vi "_TCP Msg Write_tester.vi"(7 "RT":bool, 8 "error in":errorcluster, 9 "timeout ms (10000)":i32=10000, 10 "Packet Info In":T1={"Packet Signature"="", "Sequence Number"=0, "Command"=enum."xml Set LC Input Logic", "Data Message Size"=0, "Data Message Size"="", "Data Message"="", "Error Message Size"=0, "Error Message Size"="", "Error Message"="", "Checksum"=0, "Error Message"={"status"=FALSE, "code"=0, "source"=""}, "Command ID"=""}, 11 "connection ID In":refnum<k5>) -> (0 "error out":errorcluster, 2 "Packet Info In Out":T1={"Packet Signature"="", "Sequence Number"=0, "Command"=enum."Get Info", "Data Message Size"=0, "Data Message Size"="", "Data Message"="", "Error Message Size"=0, "Error Message Size"="", "Error Message"="", "Checksum"=0, "Error Message"={"status"=FALSE, "code"=0, "source"=""}, "Command ID"=""}, 3 "connection ID out":refnum<k5>)   [LabVIEW 2015]
doc: "Writes a package of data to a remote computer via TCP/IP. The VI appends an ID number to each packet. This ID number is used by the Comm TCP Read VI to parse the packet using the meta data. This technique allows appending variable name and type to each packet for ease of use while minimizing the transmission overhead.\n\nThe data must be passed in as a String. The user is responsible for casting or flattening the desired data into a String before passing it to this VI. \n\n* Use the same method for converting to/from String on both the Read and Write functions. For example, if you use the 'Cast' primitive to convert the data into a String, make sure that the 'Cast' primitive is used on the receiving side to convert the data from String to its original form."
uses:
  Type/TCP Packet Info.ctl
  Type/_RT Command.ctl
  Type/TCP Packet Parsing State Machine.ctl
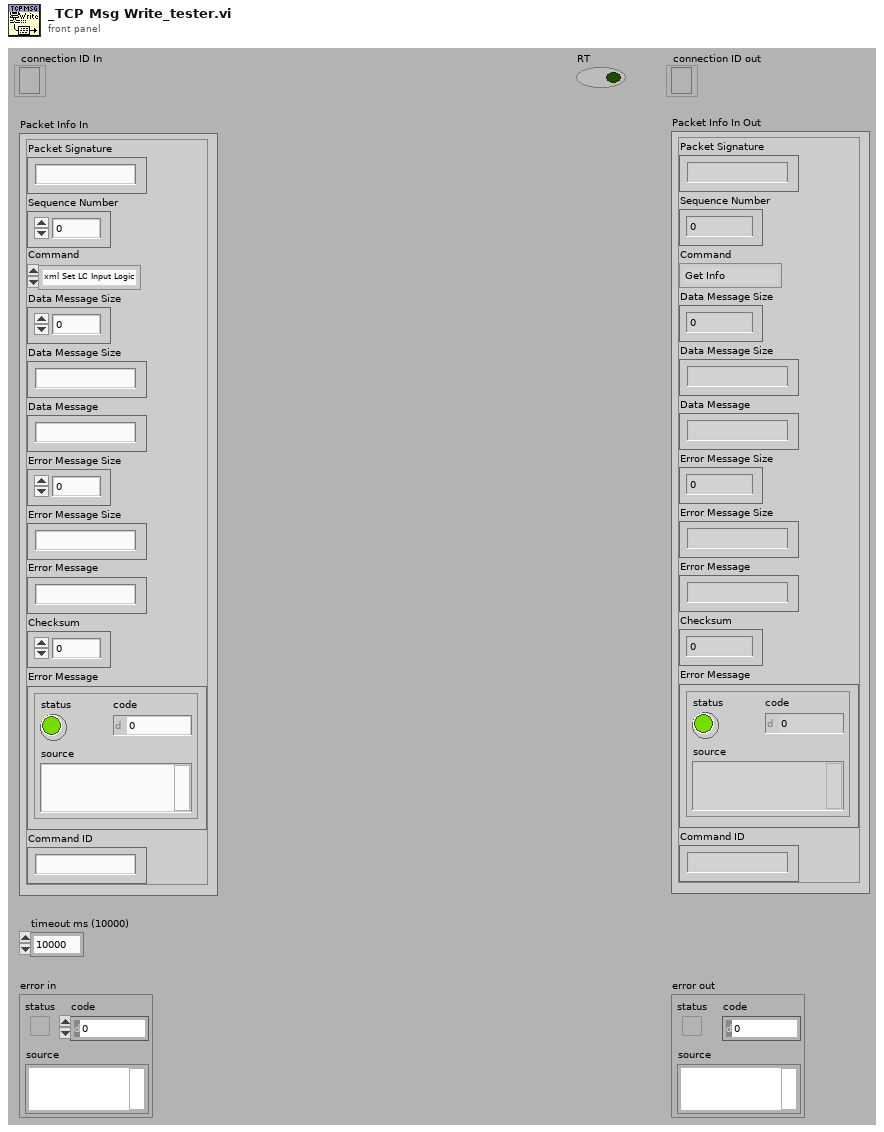
[diagram p1: front panel]
types:
  T1 = typedef "TCP Packet Info.ctl" = cluster{"Packet Signature":string, "Sequence Number":i32, "Command":T2, "Data Message Size":u32, "Data Message Size":string, "Data Message":string, "Error Message Size":u32, "Error Message Size":string, "Error Message":string, "Checksum":u32, "Error Message":errorcluster, "Command ID":string}
  T2 = typedef "_RT Command.ctl" = enum16{"xml Start Run", "xml Start Actual Run", "xml Stop Run", "xml Runtime Update", "xml Get Status", "xml Get Table", "xml Set Table", "xml Get Configuration", "xml System Status", "xml Set LC Input Logic", "xml Get Data", "xml Get Info", "Start", "StartActualRun", "Stop", "Runtime Update", "Get Data", "Get Info", "Get Status", "Get Param", "Get Config", "Get Table", "Read ADC", "Set Oscillator", "Update Config", "Update Table", "Set All Pol", "Set Pol and DC", "Set Max Mass", "Toggle RP", "Toggle EL", "Set PIC", "Initialize Turbo", "Send Turbo Comm", "Close Turbo", "P1", "P2", "P3", "Send Serial", "Set LC Out", "Get LC In", "Read VAC", "Test Table", "Toggle Power", "Get Startup", "Set Startup", "Get ADC Table", "Set ADC Table", "Get Brief Status", "Get Detail Status", "Auxiliary Update", "Set CC Logics", "Set CC Input Logics", "Ignore Error", "invalid"}
  T3 = typedef "TCP Packet Parsing State Machine.ctl" = enum16{"Packet Signature", "Sequence Number", "Command ID", "Data Message Size", "Data Message", "Error Message Size", "Error Message", "Checksum", "Invalid Packet Structure"}
  T4 = enum16{"big-endian, network order", "native, host order", "little-endian"}
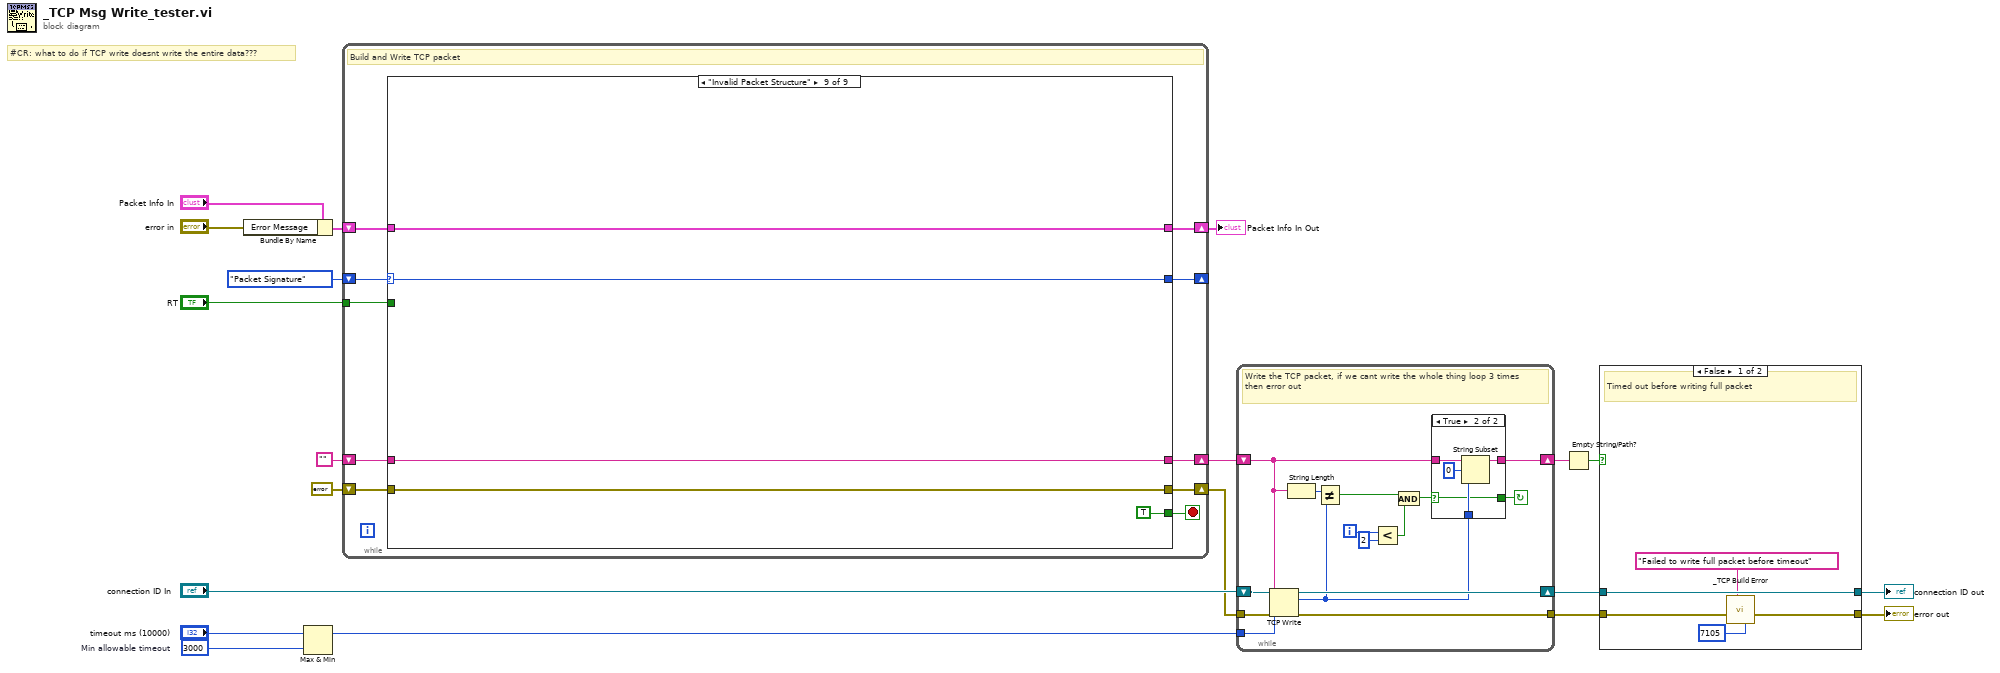
[diagram p0: block diagram]
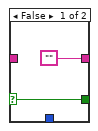
[diagram p3: hidden frame]
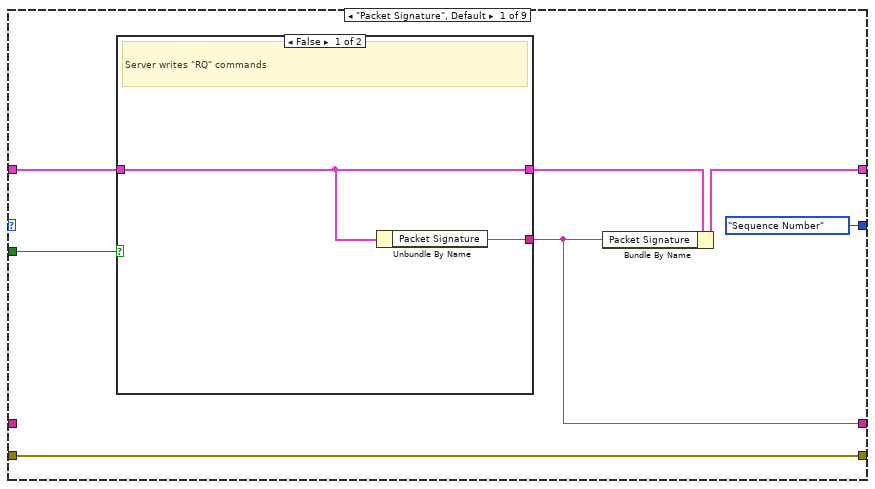
[diagram p4: hidden frame]
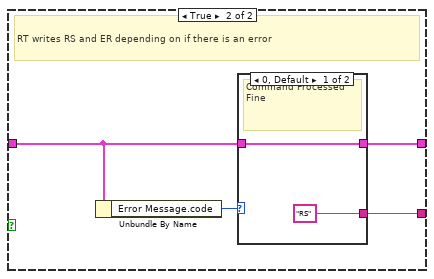
[diagram p5: hidden frame]
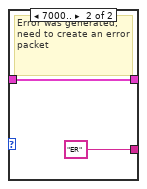
[diagram p6: hidden frame]
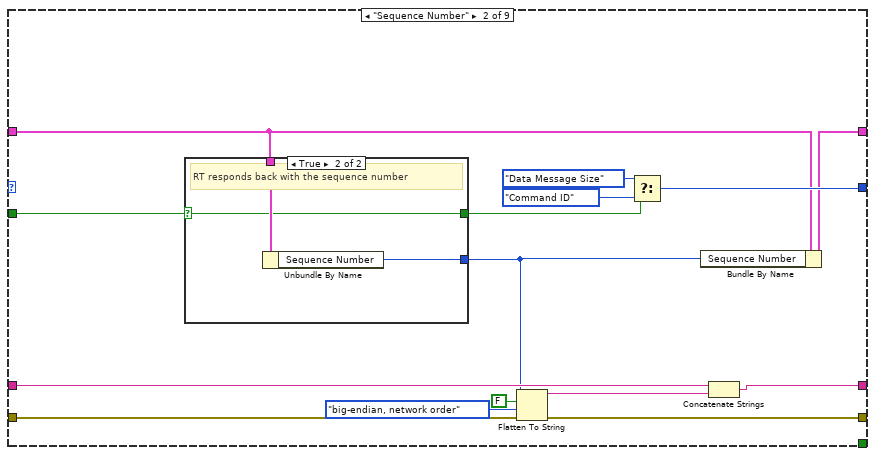
[diagram p7: hidden frame]
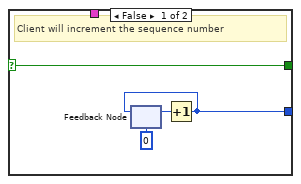
[diagram p8: hidden frame]
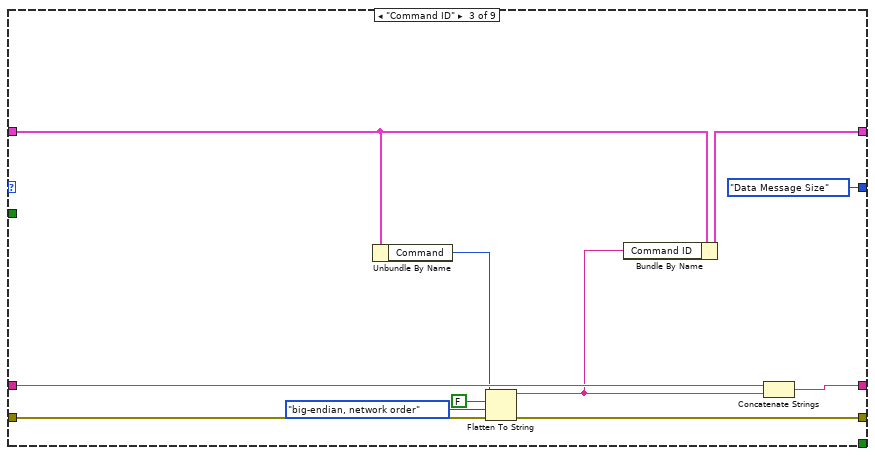
[diagram p9: hidden frame]
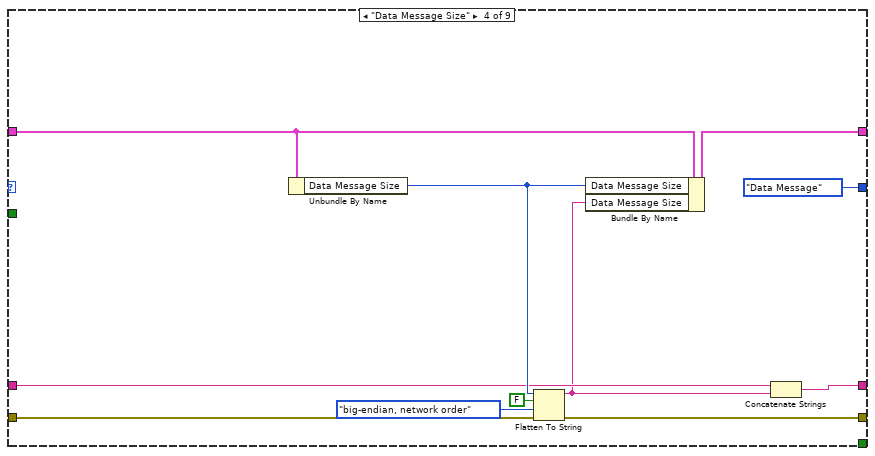
[diagram p10: hidden frame]
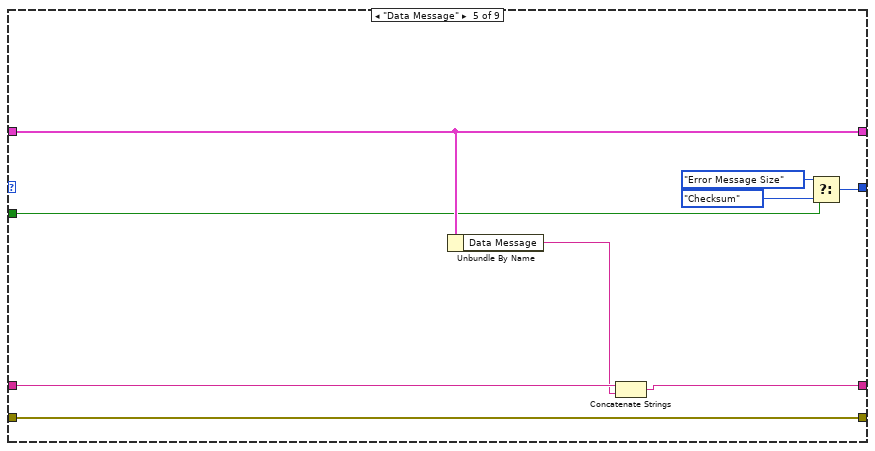
[diagram p11: hidden frame]
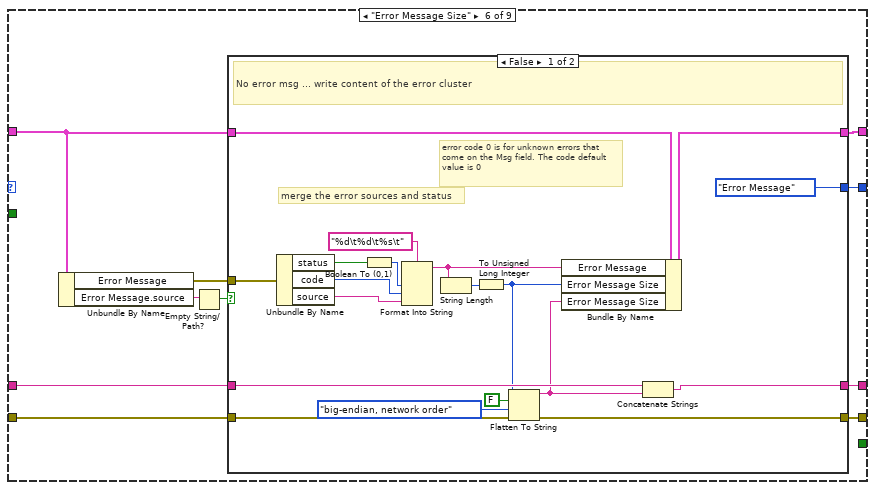
[diagram p12: hidden frame]
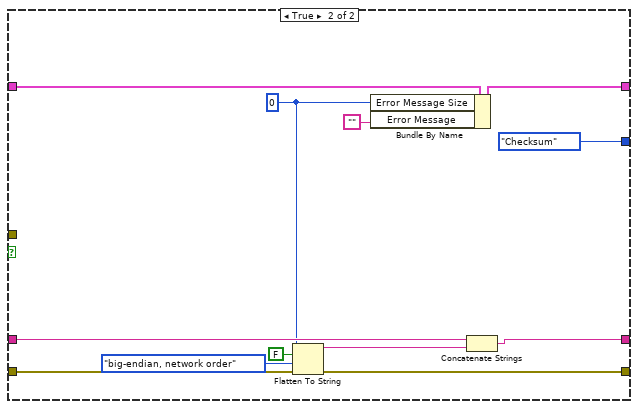
[diagram p13: hidden frame]
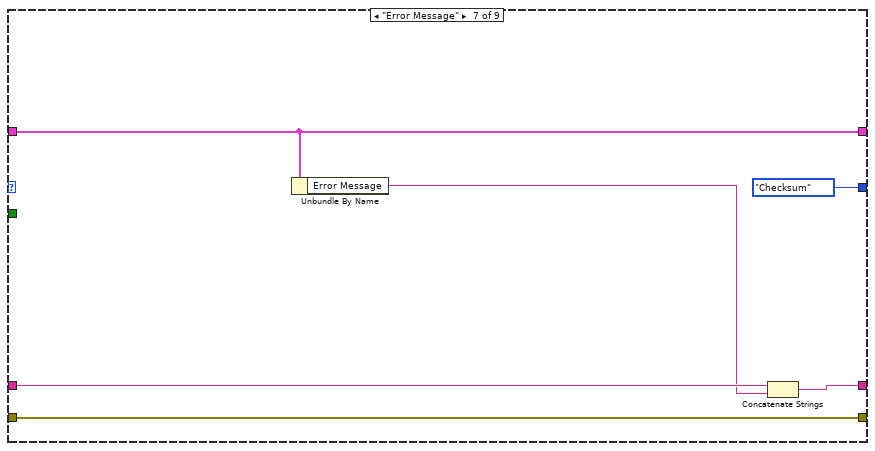
[diagram p14: hidden frame]
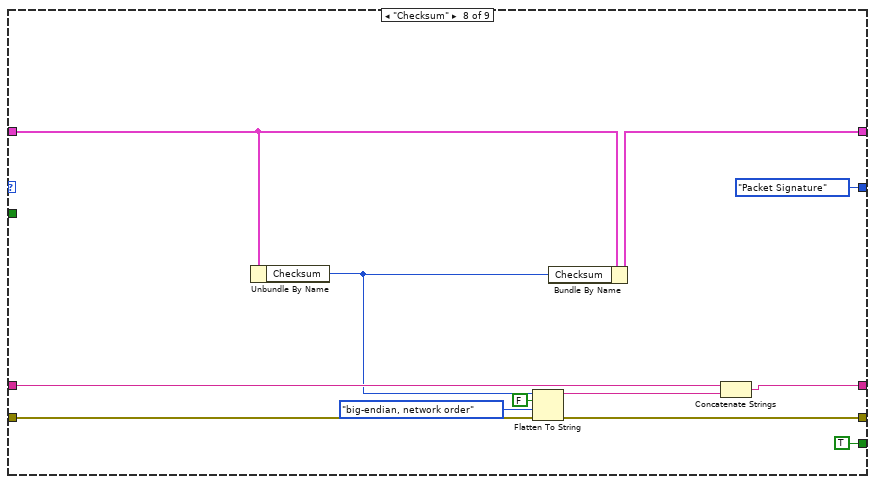
[diagram p15: hidden frame]
diagram:
  w16 = 3000  # Min allowable timeout
  # "#CR: what to do if TCP write doesnt write the entire data???"
  n1 = Bundle By Name(cluster="Packet Info In", "Error Message"="error in") -> (w15:T1)
  n2 = Max & Min(x="timeout ms (10000)", y=w16) -> (max(x,y)=w4:i32)  [unwired: 1 out]
  n3 = while {
    shift-right: [w29] -> w11
    shift-left: w15 -> [w30]
    tunnel: "RT" -> [w28]
    shift-right: [w27] -> _
    shift-left: TCP_Packet_Parsing_State_Machine."Packet Signature" ("Packet Structure") -> [w25]
    shift-right: [w23] -> w3
    shift-left: "" ("Message Packet") -> [w24]
    shift-right: [w21] -> w5
    shift-left: errorcluster {"status"=FALSE, "code"=0, "source"=""} ("error out") -> [w22]
    stop <- w26 stop-if-true
    # "Build and Write TCP packet"
    n4 = case shown="\"Invalid Packet Structure\"" w25 {
      selector: w25 -> [_ _ _ _ _ _ _ _ w162]
      tunnel: w30 -> [w35 w58 w80 w90 w100 w105 w147 w158 w164]
      tunnel: [w32 w49 w71 w82 w100 w106 w147 w159 w164] -> w29
      tunnel: w28 -> [w37 w59 _ _ w98 _ _ _ _]
      tunnel: [TCP_Packet_Parsing_State_Machine."Sequence Number" ("Packet Structure") w61 TCP_Packet_Parsing_State_Machine."Data Message Size" ("Packet Structure") TCP_Packet_Parsing_State_Machine."Data Message" ("Packet Structure") w99 w109 TCP_Packet_Parsing_State_Machine."Checksum" ("Packet Structure") TCP_Packet_Parsing_State_Machine."Packet Signature" ("Packet Structure") w162] -> w27
      tunnel: [_ _ _ _ _ _ _ TRUE TRUE] -> w26
      tunnel: w24 -> [_ w56 w78 w87 w95 w104 w145 w155 w161]
      tunnel: [w31 w55 w77 w88 w94 w103 w144 w154 w161] -> w23
      tunnel: w22 -> [w33 w54 w74 w83 w92 w101 w142 w149 w160]
      tunnel: [w33 w51 w73 w84 w92 w102 w142 w151 w160] -> w21
      frame "Packet Signature", Default {
        # "Packet Header"
        n5 = case shown="False" w37 {
          tunnel: w35 -> [w39 w43]
          tunnel: [w39 w42] -> w36
          tunnel: [w38 w41] -> w31
          frame False {
            # "Server writes \"RQ\" commands"
            n6 = Unbundle By Name(w39) -> ("Packet Signature"=w38:string)
          }
          frame True {
            # "RT writes RS and ER depending on if there is an error"
            n7 = Unbundle By Name(w43) -> ("Error Message.code"=w40:i32)
            n8 = case shown="0, Default" w40 {
              tunnel: w43 -> [w45 w47]
              tunnel: [w45 w47] -> w42
              tunnel: ["RS" ("data in") "ER" ("data in")] -> w41
              frame 0, Default {
                # "Command Processed Fine"
              }
              frame 7000.. {
                # "Error was generated, need to create an error packet"
              }
            }
          }
        }
        n9 = Bundle By Name(cluster=w36, "Packet Signature"=w31) -> (w32:T1)
      }
      frame "Sequence Number" {
        n10 = case shown="True" w59 {
          selector: w59 -> [w63 w67]
          tunnel: w58 -> [_ w69]
          tunnel: [w64 w68] -> w48
          tunnel: [w63 w67] -> w57
          frame False {
            # "Client will increment the sequence number"
            n11 = feedback #1(0 ("Sequence Number")) -> (w65:i32)
            n12 = Increment(x=w65) -> (x+1=w64:i32)
            n13 = feedback-in #1(w64) -> ()
          }
          frame True {
            # "RT responds back with the sequence number"
            n14 = Unbundle By Name(w69) -> ("Sequence Number"=w68:i32)
          }
        }
        n15 = Flatten To String(anything=w48, prepend array or string size? (T)=FALSE, byte order (0:big-endian, network order)=T4."big-endian, network order", error in (no error)=w54) -> (data string=w52:string, error out=w51:errorcluster)  [unwired: 1 out]
        n16 = Select(t=TCP_Packet_Parsing_State_Machine."Data Message Size" ("Packet Structure"), s=w57, f=TCP_Packet_Parsing_State_Machine."Command ID") -> (s? t:f=w61:T3)
        n17 = Bundle By Name(cluster=w58, "Sequence Number"=w48) -> (w49:T1)
        n18 = Concatenate Strings(w56, w52) -> (w55:string)
      }
      frame "Command ID" {
        n19 = Unbundle By Name(w80) -> ("Command"=w72:T2)
        n20 = Flatten To String(anything=w72, prepend array or string size? (T)=FALSE, byte order (0:big-endian, network order)=T4."big-endian, network order", error in (no error)=w74) -> (data string=w70:string, error out=w73:errorcluster)  [unwired: 1 out]
        n21 = Bundle By Name(cluster=w80, "Command ID"=w70) -> (w71:T1)
        n22 = Concatenate Strings(w78, w70) -> (w77:string)
      }
      frame "Data Message Size" {
        n23 = Unbundle By Name(w90) -> ("Data Message Size"=w89:u32)
        n24 = Flatten To String(anything=w89, prepend array or string size? (T)=FALSE ("data includes array or string size? (T)"), byte order (0:big-endian, network order)=T4."big-endian, network order", error in (no error)=w83) -> (data string=w81:string, error out=w84:errorcluster)  [unwired: 1 out]
        n25 = Bundle By Name(cluster=w90, "Data Message Size"=w89, "Data Message Size"=w81) -> (w82:T1)
        n26 = Concatenate Strings(w87, w81) -> (w88:string)
      }
      frame "Data Message" {
        n27 = Unbundle By Name(w100) -> ("Data Message"=w93:string)
        n28 = Concatenate Strings(w95, w93) -> (w94:string)
        n29 = Select(t=TCP_Packet_Parsing_State_Machine."Error Message Size" ("f"), s=w98, f=TCP_Packet_Parsing_State_Machine."Checksum" ("Packet Structure")) -> (s? t:f=w99:T3)
      }
      frame "Error Message Size" {
        n30 = Unbundle By Name(w105) -> ("Error Message"=w108:errorcluster, "Error Message.source"=w107:string)
        n31 = Empty String/Path?(string/path=w107) -> (empty?=w110:bool)
        n32 = case shown="False" w110 {
          tunnel: [TCP_Packet_Parsing_State_Machine."Error Message" ("Packet Structure") TCP_Packet_Parsing_State_Machine."Checksum" ("Packet Structure")] -> w109
          tunnel: w108 -> [w128 _]
          tunnel: [w122 w133] -> w106
          tunnel: w105 -> [w123 w140]
          tunnel: w104 -> [w118 w135]
          tunnel: [w117 w134] -> w103
          tunnel: [w115 w136] -> w102
          tunnel: w101 -> [w114 w137]
          frame False {
            # "error code 0 is for unknown errors that \ncome on the Msg field. The code default \nvalue is 0"
            # "merge the error sources and status"
            # "No error msg ... write content of the error cluster"
            n33 = Unbundle By Name(w128) -> ("status"=w119:bool, "code"=w125:i32, "source"=w124:string)
            n34 = Boolean To (0,1)(Boolean=w119) -> (0, 1=w126:i16)
            n35 = Format Into String(format string="%d\t%d\t%s\t", w126, w125, w124) -> (resulting string=w121:string)  [unwired: 2 in, 1 out]
            n36 = String Length(string=w121) -> (length=w120:i32)
            n37 = To Unsigned Long Integer(number=w120) -> (unsigned 32bit integer=w112:u32)
            n38 = Flatten To String(anything=w112, prepend array or string size? (T)=FALSE ("data includes array or string size? (T)"), byte order (0:big-endian, network order)=T4."big-endian, network order", error in (no error)=w114) -> (data string=w111:string, error out=w115:errorcluster)  [unwired: 1 out]
            n39 = Bundle By Name(cluster=w123, "Error Message"=w121, "Error Message Size"=w112, "Error Message Size"=w111) -> (w122:T1)
            n40 = Concatenate Strings(w118, w111) -> (w117:string)
          }
          frame True {
            w132 = u32 0 ("unsigned 32bit integer")
            n41 = Flatten To String(anything=w132, prepend array or string size? (T)=FALSE ("data includes array or string size? (T)"), byte order (0:big-endian, network order)=T4."big-endian, network order", error in (no error)=w137) -> (data string=w131:string, error out=w136:errorcluster)  [unwired: 1 out]
            n42 = Bundle By Name(cluster=w140, "Error Message Size"=w132, "Error Message"="") -> (w133:T1)
            n43 = Concatenate Strings(w135, w131) -> (w134:string)
          }
        }
      }
      frame "Error Message" {
        n44 = Unbundle By Name(w147) -> ("Error Message"=w143:string)
        n45 = Concatenate Strings(w145, w143) -> (w144:string)
      }
      frame "Checksum" {
        n46 = Unbundle By Name(w158) -> ("Checksum"=w148:u32)
        n47 = Flatten To String(anything=w148, prepend array or string size? (T)=FALSE ("data includes array or string size? (T)"), byte order (0:big-endian, network order)=T4."big-endian, network order", error in (no error)=w149) -> (data string=w150:string, error out=w151:errorcluster)  [unwired: 1 out]
        n48 = Bundle By Name(cluster=w158, "Checksum"=w148) -> (w159:T1)
        n49 = Concatenate Strings(w155, w150) -> (w154:string)
      }
      frame "Invalid Packet Structure" {
      }
    }
  }
  "Packet Info In Out" <- w11
  n50 = while {
    tunnel: w4 -> [w176]
    shift-right: [w179] -> w10
    shift-left: "connection ID In" -> [w177]
    shift-right: [w174] -> w2
    shift-left: w3 -> [w172]
    tunnel: w5 -> [w175]
    tunnel: [w178] -> w9
    i -> [w169]
    stop <- w173 continue-if-true
    # "Write the TCP packet, if we cant write the whole thing loop 3 times then error out"
    n51 = TCP Write(connection ID=w177, data in=w172, error in (no error)=w175, 9:w176) -> (connection ID out=w179:refnum<k5>, bytes written=w170:i32, error out=w178:errorcluster)
    n52 = String Length(string=w172) -> (length=w171:i32)
    n53 = Not Equal?(x=w171, y=w170) -> (x != y?=w167:bool)
    n54 = Less?(x=w169, y=2) -> (x < y?=w165:bool)
    n55 = And(x=w167, y=w165) -> (x .and. y?=w166:bool)
    n56 = case shown="True" w166 {
      selector: w166 -> [w181 w182]
      tunnel: ["" w183] -> w174
      tunnel: w172 -> [_ w184]
      tunnel: [w181 w182] -> w173
      tunnel: w170 -> [_ w185]
      frame False {
      }
      frame True {
        n57 = String Subset(string=w184, offset (0)=0, length (rest)=w185) -> (substring=w183:string)
      }
    }
  }
  n58 = Empty String/Path?(string/path=w2) -> (empty?=w1:bool)
  n59 = case shown="False" w1 {
    tunnel: w9 -> [w190 w192]
    tunnel: [w191 w193] -> w8
    tunnel: w10 -> [w191 w193]
    tunnel: [w189 w192] -> w7
    frame False {
      # "Timed out before writing full packet"
      n60 = call "_TCP Build Error.vi"("code"=7105, "Error"="Failed to write full packet before timeout", "error in (no error)"=w190) -> ("error out"=w189:errorcluster)  [unwired: 8 in]
    }
    frame True {
      # "everything was written"
    }
  }
  "error out" <- w7
  "connection ID out" <- w8
